vi "Kinesis - KDC101 - No Front Panel_mod.vi"() -> ()   [LabVIEW 2019]
uses:
  C:/Program Files (x86)/National Instruments/LabVIEW 2019/user.lib/ThorKDC101/Kinesis_with_LabVIEW_Examples_LV12 - v3/Thorlabs.MotionControl.DeviceManagerCLI.dll
  Thorlabs.MotionControl.DeviceManagerCLI.dll
  C:/Program Files (x86)/National Instruments/LabVIEW 2019/user.lib/ThorKDC101/Kinesis_with_LabVIEW_Examples_LV12 - v3/ThorLabs.MotionControl.KCube.DCServoCLI.dll
  ThorLabs.MotionControl.KCube.DCServoCLI.dll
  C:/Program Files (x86)/National Instruments/LabVIEW 2019/user.lib/ThorKDC101/Kinesis_with_LabVIEW_Examples_LV12 - v3/Thorlabs.MotionControl.GenericMotorCLI.dll
  Thorlabs.MotionControl.GenericMotorCLI.dll
panel:
  out "IsHomed":bool
  out "MinVelocity":dbl
  out "MaxVelocity":dbl
  out "Acceleration":dbl
  out "x/y":dbl
  out "DevicePosition":i32
  out "Position":i64
  out "GetPositionCounter":i32
  out "GetMoveAbsolutePosition":dbl
  out "Count":i32
  out "Capacity":i32
  out "array":string[](array[string])=["", "", "", "", "", "", "", "", "", "", " "]
  out "Moving":bool
  out "Controller Information":T1
  in  "Type the name of the Stage/Actuator e.g. MTS50/M-Z8":string
  in  "serialNo":string
  # "Thorlabs Hardware: KDC101 - K-Cube Brushed DC Servo Motor Controller\n https://www.thorlabs.com/thorproduct.cfm?partnumber=KDC101\n\nDescription: This VI is an example of communicating with Thorlabs Motion Control devices outside of the provided WinForms UI controls contained in Thorlabs.MotionControl.Controls.dll.\nInstead, we introduce how you can make use of the wider range of Generic & Device-specific component DLLs included with your Kinesis Installation. \n\nThe VI will identify & connect to your KDC101 through BuildDeviceList() & assign Motor Settings based on the actuator/stage name entered into the control detailed in the ThorlabsDefaultSettings file. \nDevice information will output to the 'Controller Information' cluster & then he connected device will perform a 'Home'. A Virtual Boolean LED will identify whether the device is moving & will end the program when the device is 'Homed'.\n\nInstructions: \n1) Connect your KDC101 device to your PC & power the device, ensuring your stage/actutator is connected. For full device setup, \nthe device product manual can be found on our website here. - https://www.thorlabs.com/thorproduct.cfm?partnumber=KDC101\n2) Enter the device serial number & actuator/stage name to the left. To ensure the correct string is used, you can copy your Stage/Actuator Part Number from ThorlabsDefaultSettings file found in: \nC:\\Program Files (x86)\\Thorlabs\\Kinesis or\nC:\\Program Files\\Thorlabs\\Kinesis\n\n3) Click 'Run' in the LabVIEW Toolbar."
  # "Notes:"
  # "- Open the example VI through the LabVIEW Project Explorer to correctly load the dlls.\n\n\n\n\n\n\n\n\n\n\n\n\n- To explore the range of methods available, please visit the .NET API, included with your Kinesis software.\n\n- For tips on building your own VIs with Thorlabs Motion Control Hardware, please see our LabVIEW Guide here.\nhttps://www.thorlabs.com/newgrouppage9.cfm?objectgroup_id=10285"
  # "- Ensure that the appropriate .DLLs are copied into your Project Folder. Check that the correct bit type are used depending on your version of LabVIEW\ni.e. 32-bit or 64-bit."
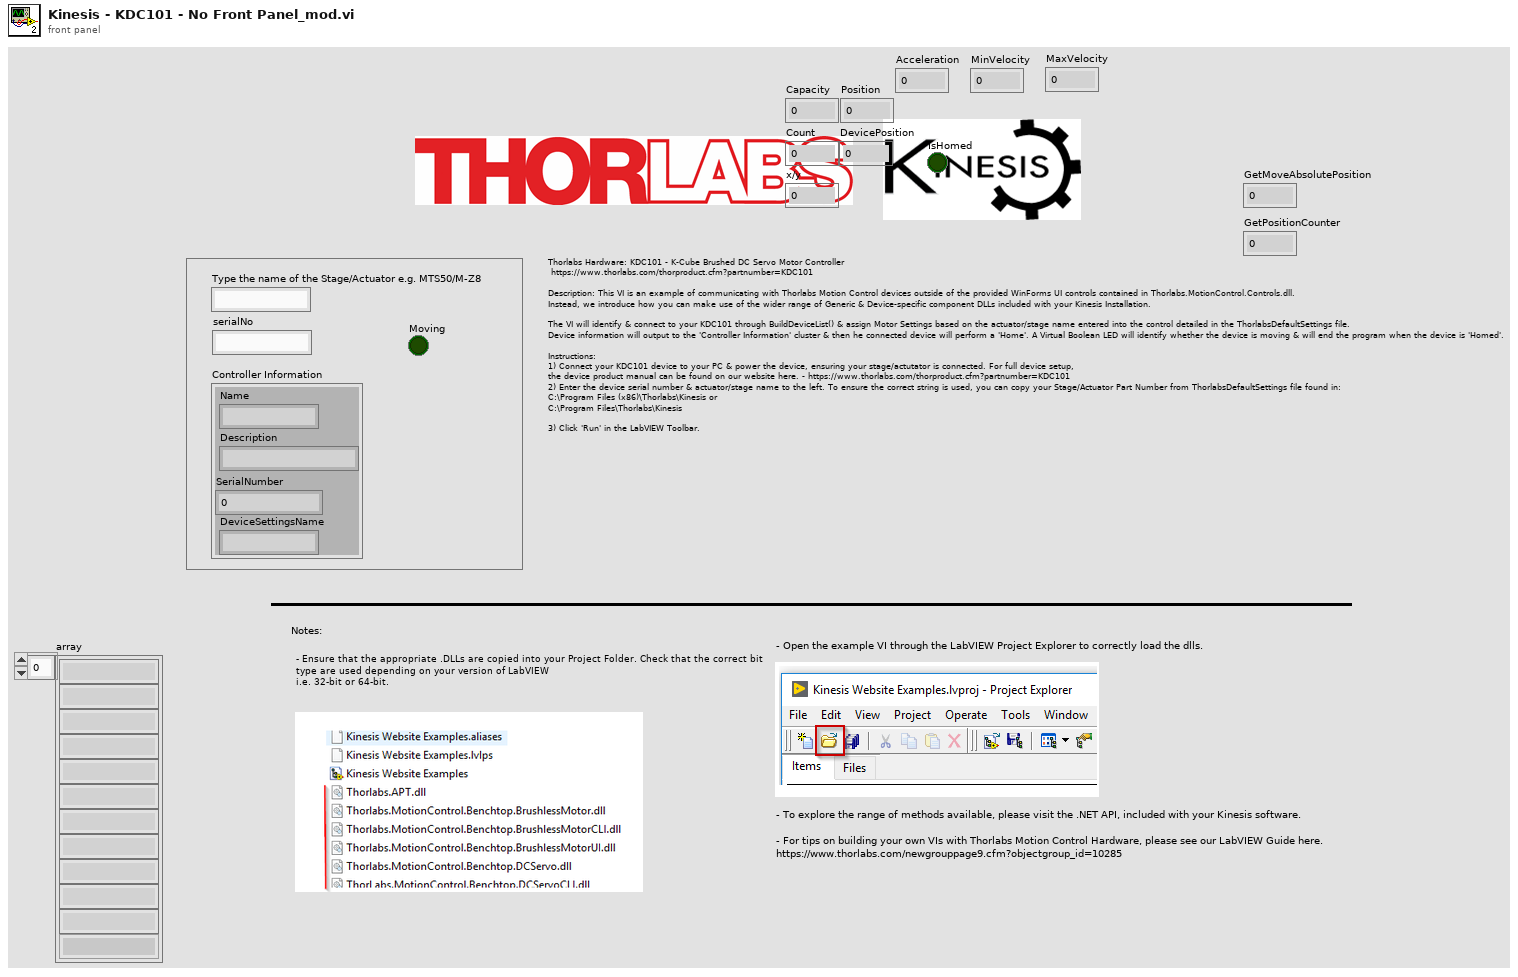
[diagram p1: front panel]
types:
  T1 = cluster{"Name":string, "Description":string, "SerialNumber":u32, "DeviceSettingsName":string}
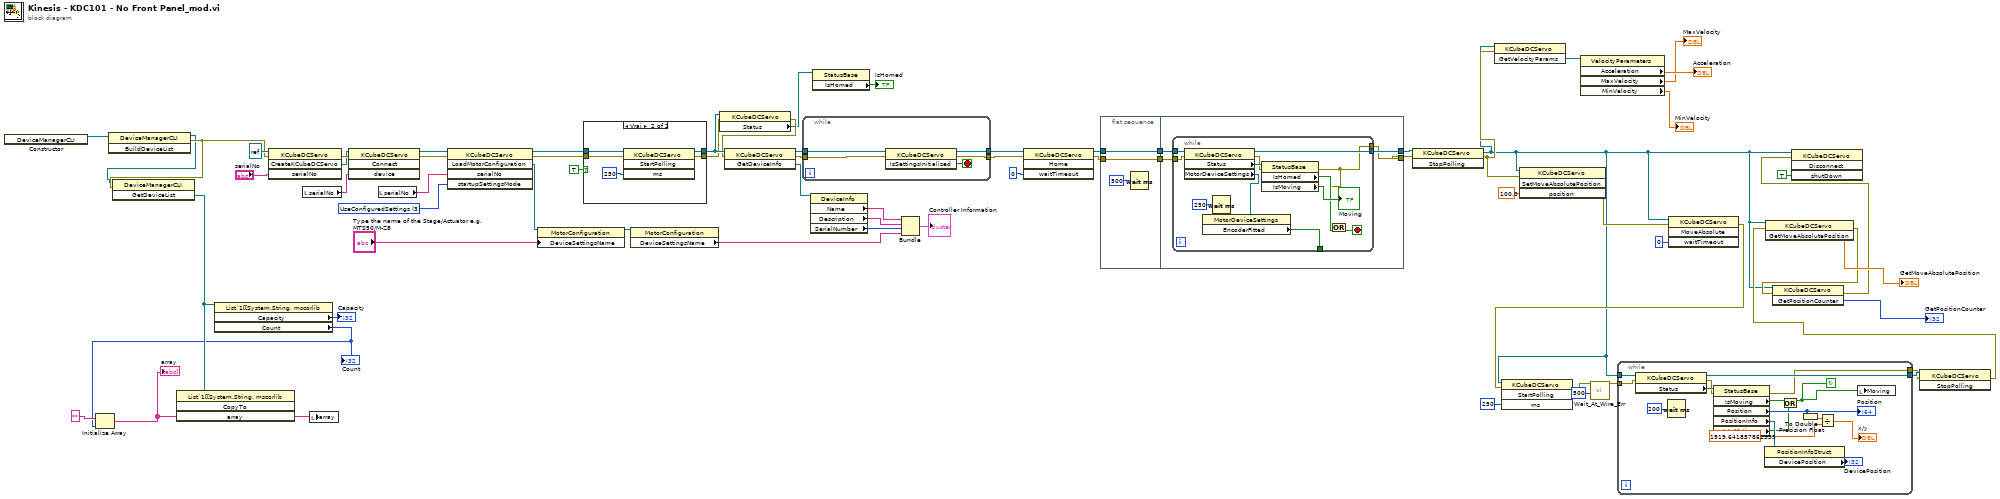
[diagram p0: block diagram]
diagram:
  w49 = 3 items=["UseDeviceSettings"=1, "UseFileSettings"=2, "UseConfiguredSettings"=3] ("startupSettingsMode")
  n1 = constructor class="DeviceManagerCLI"() -> (reference out=w39:refnum<k24>)  [unwired: 3 in, 2 out]
  n2 = invoke class="DeviceManagerCLI" method="BuildDeviceList"(reference=w39) -> (reference out=w34:refnum<k24>, error out=w35:errorcluster)  [unwired: 2 in, 1 out]
  n3 = invoke class="DeviceManagerCLI" method="GetDeviceList"(reference=w34, error in=w35) -> ("GetDeviceList"=w32:refnum<k24>)  [unwired: 1 in, 2 out]
  n4 = property class="List`1[[System.String, mscorlib"(reference=w32) -> ("Capacity"=→"Capacity":i32, "Count"=w29:i32)  [unwired: 1 in, 2 out]
  "Count" <- w29
  n5 = Initialize Array("", w29) -> (w28:string[])
  "array" <- w28
  n6 = invoke class="List`1[[System.String, mscorlib" method="CopyTo"(reference=w32, "array"=w28) -> ("array"=w33:string[])  [unwired: 2 in, 3 out]
  n7 = invoke class="KCubeDCServo" method="CreateKCubeDCServo"(reference=refnum<k24> refnum ("target class"), error in=w35, "serialNo"="serialNo") -> (error out=w67:errorcluster, "CreateKCubeDCServo"=w64:refnum<k24>)  [unwired: 1 in, 2 out]
  n8 = local read "serialNo"() -> (w66:string)
  n9 = local write "array"(w33) -> ()
  n10 = invoke class="KCubeDCServo" method="Connect"(reference=w64, error in=w67, "device"=w66) -> (reference out=w47:refnum<k24>, error out=w45:errorcluster)  [unwired: 1 in, 2 out]
  n11 = local read "serialNo"() -> (w46:string)
  n12 = invoke class="KCubeDCServo" method="LoadMotorConfiguration"(reference=w47, error in=w45, "serialNo"=w46, "startupSettingsMode"=w49) -> (reference out=w62:refnum<k24>, error out=w44:errorcluster, "LoadMotorConfiguration"=w56:refnum<k24>)  [unwired: 1 in, 2 out]
  n13 = property class="MotorConfiguration"(reference=w56, "DeviceSettingsName"="Type the name of the Stage/Actuator e.g. MTS50/M-Z8") -> (reference out=w58:refnum<k24>)  [unwired: 1 in, 1 out]
  n14 = case shown="Vrai" TRUE {
    tunnel: w62 -> [w69 w75]
    tunnel: [w69 w74] -> w5
    tunnel: w44 -> [w70 w72]
    tunnel: [w70 w71] -> w4
    frame False {
    }
    frame True {
      n15 = invoke class="KCubeDCServo" method="StartPolling"(reference=w75, error in=w72, "ms"=250) -> (reference out=w74:refnum<k24>, error out=w71:errorcluster)  [unwired: 1 in, 2 out]
    }
  }
  n16 = property class="MotorConfiguration"(reference=w58) -> ("DeviceSettingsName"=w59:string)  [unwired: 1 in, 2 out]
  n17 = property class="KCubeDCServo"(reference=w5, error in=w4) -> (error out=w3:errorcluster, "Status"=w2:refnum<k24>)  [unwired: 1 out]
  n18 = invoke class="KCubeDCServo" method="GetDeviceInfo"(reference=w5, error in=w3) -> (reference out=w52:refnum<k24>, error out=w43:errorcluster, "GetDeviceInfo"=w51:refnum<k24>)  [unwired: 1 in]
  n19 = while {
    tunnel: [w79] -> w50
    tunnel: w52 -> [w80]
    tunnel: w43 -> [w77]
    tunnel: [w76] -> w42
    stop <- w78 stop-if-true
    n20 = invoke class="KCubeDCServo" method="IsSettingsInitialized"(reference=w80, error in=w77) -> (reference out=w79:refnum<k24>, error out=w76:errorcluster, "IsSettingsInitialized"=w78:bool)  [unwired: 1 in]
  }
  n21 = property class="DeviceInfo"(reference=w51) -> ("Name"=w53:string, "Description"=w54:string, "SerialNumber"=w55:u32)  [unwired: 1 in, 2 out]
  n22 = property class="StatusBase"(reference=w2) -> ("IsHomed"=→"IsHomed":bool)  [unwired: 1 in, 2 out]
  n23 = Bundle("Name"=w53, "Description"=w54, "SerialNumber"=w55, "DeviceSettingsName"=w59) -> (→"Controller Information":T1)  [unwired: 1 in]
  n24 = invoke class="KCubeDCServo" method="Home"(reference=w50, error in=w42, "waitTimeout"=0) -> (reference out=w61:refnum<k24>, error out=w40:errorcluster)  [unwired: 1 in, 2 out]
  n25 = flat-sequence {
    tunnel: [w83] -> w63
    tunnel: w61 -> [w83]
    tunnel: [w82] -> w41
    tunnel: w40 -> [w82]
    tunnel: [w87] -> w38
    tunnel: w63 -> [w86]
    tunnel: w41 -> [w85]
    tunnel: [w84] -> w37
    frame #0 {
      n26 = Wait (ms)(milliseconds to wait=u32 500) -> ()  [unwired: 1 out]
    }
    frame #1 {
      n27 = while {
        tunnel: [w96] -> w87
        tunnel: w86 -> [w97]
        tunnel: w85 -> [w94]
        tunnel: [w90] -> w84
        tunnel: [w88] -> _
        stop <- w91 stop-if-true
        n28 = property class="KCubeDCServo"(reference=w97, error in=w94) -> (reference out=w96:refnum<k24>, error out=w93:errorcluster, "Status"=w98:refnum<k24>, "MotorDeviceSettings"=w89:refnum<k24>)
        n29 = property class="MotorDeviceSettings"(reference=w89) -> ("EncoderFitted"=w88:bool)  [unwired: 1 in, 2 out]
        n30 = Wait (ms)(milliseconds to wait=u32 250) -> ()  [unwired: 1 out]
        n31 = property class="StatusBase"(reference=w98, error in=w93) -> (error out=w90:errorcluster, "IsHomed"=w95:bool, "IsMoving"=→"Moving":bool)  [unwired: 1 out]
        n32 = Or(x=w90, y=w95) -> (x .or. y?=w91:bool)
      }
    }
  }
  n33 = invoke class="KCubeDCServo" method="StopPolling"(reference=w38, error in=w37) -> (reference out=w6:refnum<k24>, error out=w11:errorcluster)  [unwired: 1 in, 1 out]
  n34 = invoke class="KCubeDCServo" method="GetVelocityParams"(reference=w6, error in=w11) -> ("GetVelocityParams"=w10:refnum<k24>)  [unwired: 1 in, 2 out]
  n35 = invoke class="KCubeDCServo" method="SetMoveAbsolutePosition"(reference=w6, error in=w11, "position"=100.0) -> (error out=w26:errorcluster)  [unwired: 1 in, 3 out]
  n36 = property class="VelocityParameters"(reference=w10) -> ("Acceleration"=→"Acceleration":dbl, "MaxVelocity"=→"MaxVelocity":dbl, "MinVelocity"=→"MinVelocity":dbl)  [unwired: 1 in, 2 out]
  n37 = invoke class="KCubeDCServo" method="MoveAbsolute"(reference=w6, error in=w26, "waitTimeout"=0) -> (error out=w19:errorcluster)  [unwired: 1 in, 3 out]
  n38 = invoke class="KCubeDCServo" method="StartPolling"(reference=w6, error in=w19, "ms"=250) -> (error out=w14:errorcluster)  [unwired: 1 in, 3 out]
  n39 = call <userlib>:"Wait_At_Wire_Err.vi"("Wait (ms)"=u32 500, "error in (no error)"=w14) -> ("error out"=w13:errorcluster)  [unwired: 7 in, 2 out]
  n40 = while {
    tunnel: [w113] -> w18
    tunnel: w6 -> [w114]
    tunnel: w13 -> [w112]
    tunnel: [w110] -> w16
    stop <- w101 continue-if-true
    n41 = property class="KCubeDCServo"(reference=w114, error in=w112) -> (reference out=w113:refnum<k24>, error out=w111:errorcluster, "Status"=w115:refnum<k24>)
    n42 = Wait (ms)(milliseconds to wait=u32 200) -> ()  [unwired: 1 out]
    n43 = property class="StatusBase"(reference=w115, error in=w111) -> (error out=w110:errorcluster, "IsMoving"=w109:bool, "Position"=w104:i64, "PositionInfo"=w107:refnum<k24>, "IsInMotion"=w100:bool)  [unwired: 1 out]
    "Position" <- w104
    n44 = property class="PositionInfoStruct"(reference=w107) -> ("DevicePosition"=→"DevicePosition":i32)  [unwired: 1 in, 2 out]
    n45 = Or(x=w109, y=w100) -> (x .or. y?=w101:bool)
    n46 = To Double Precision Float(number=w104) -> (double precision float=w102:dbl)
    n47 = Divide(x=w102, y=1919.641857862339) -> (x/y=→"x/y":dbl)
    n48 = local write "Moving"(w101) -> ()
  }
  n49 = invoke class="KCubeDCServo" method="StopPolling"(reference=w18, error in=w16) -> (error out=w17:errorcluster)  [unwired: 1 in, 2 out]
  n50 = invoke class="KCubeDCServo" method="GetMoveAbsolutePosition"(reference=w6, error in=w17) -> (error out=w23:errorcluster, "GetMoveAbsolutePosition"=→"GetMoveAbsolutePosition":dbl)  [unwired: 1 in, 1 out]
  n51 = invoke class="KCubeDCServo" method="GetPositionCounter"(reference=w6, error in=w23) -> (error out=w22:errorcluster, "GetPositionCounter"=→"GetPositionCounter":i32)  [unwired: 1 in, 1 out]
  n52 = invoke class="KCubeDCServo" method="Disconnect"(reference=w6, error in=w22, "shutDown"=TRUE) -> ()  [unwired: 1 in, 4 out]
